vi "Read enabled channels.vi"(11 "niUSRP Stream Control (DMA) v1 FPGA in":refnum<class "niUSRP Stream Control (DMA) v1 FPGA.lvclass">) -> (2 "enabled channels":u32, 3 "niUSRP Stream Control (DMA) v1 FPGA out":refnum<class "niUSRP Stream Control (DMA) v1 FPGA.lvclass">)   [LabVIEW 2025, in "niUSRP Stream Control (DMA) v1 FPGA.lvclass"]
uses:
  niUSRP Stream Control (DMA) v1 FPGA.lvclass
  niUSRP Stream Control (DMA) v1 FPGA.lvclass/niUSRP Stream Control (DMA) v1 FPGA.ctl
  <vilib>/rvi/DataTransferAndStorage/Container/Common/niFpgaContainerExecOnDevCompGetState.vi
  <vilib>/rvi/Emulation/niFpgaEmulationIsFPGAContextNoSignature.vi
  <vilib>/rvi/DataTransferAndStorage/Container/Common/niFpgaContainerGetUniqueNameForEmu.vi
  <vilib>/rvi/Memory/Memory_Emulation/niFpgaMemoryEmulationCacheClearOnFirstRun.vi
  <vilib>/rvi/Memory/Memory_Emulation/nirvimemoryEmulationManagerCache_MakeExclusive.vi
  <vilib>/rvi/Memory/Memory_Emulation/niFpgaMemoryEmulationValidateCache.vi
  <vilib>/rvi/Memory/Memory_Emulation/nirvimemoryEmulationManagerCache_InsertValue.vi
  <vilib>/Utility/error.llb/Clear Errors.vi
  <vilib>/rvi/Memory/Memory_Emulation/nirvimemoryEmulationManagerCache_ReleaseExclusive.vi
  <vilib>/rvi/Memory/Memory_Emulation/nirvimemoryEmulationManagerCache_GetValue.vi
  <vilib>/rvi/Memory/Memory_Emulation/nirvimemoryEmulationManagerCache_SetValue.vi
  <vilib>/rvi/Emulation/niFpgaProcessEmulError.vi
  <vilib>/rvi/Emulation/niFpgaSctlEmulationGetInTimedLoop.vi
  <vilib>/rvi/DataTransferAndStorage/Container/XNode/niFpgaContainer.xnode
  <vilib>/rvi/DataTransferAndStorage/Register/Emulation/niFpgaRegisterEmulationRefIn.vi
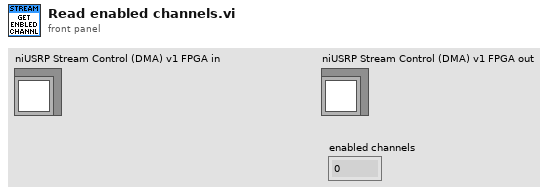
[diagram p1: front panel]
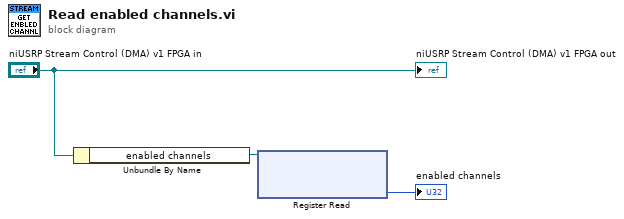
[diagram p0: block diagram]
diagram:
  n1 = Unbundle By Name("niUSRP Stream Control (DMA) v1 FPGA in") -> ("enabled channels"=w2:refnum<k21>)
  n2 = xnode "Register Read"("Register In"=w2) -> ("Data"=→"enabled channels":u32)  [unwired: 1 out]
  "niUSRP Stream Control (DMA) v1 FPGA out" <- "niUSRP Stream Control (DMA) v1 FPGA in"
